vi "EFDUV Example Read Ultimus V Dispense Parameters.vi"(0 "VISA resource name":refnum<visa-resource-name>="COM1", 5 "Serial Configuration":T1={"Baud Rate "=115200, "Parity "=0, "Data Bits "=8, "Stop Bits"=10} {"Stop Bits" items=["1.0"=10, "1.5"=15, "2.0"=20]; "Data Bits" items=["7"=7, "8"=8]; "Parity" items=["None", "Odd", "Even"]; "Baud Rate" items=["9600"=9600, "19200"=19200, "38400"=38400, "115200"=115200]}) -> (1 "CLOCK":string caption="Start", 2 "SHOT":i32 caption="Start" format="%07.0f", 3 "TRIGGER":dbl caption="Start", 4 "START":i32 caption="Start", 6 "END":i32 caption="Start", 8 "STEADY LABEL":string caption="Start", 10 "PRES":dbl caption="Start", 12 "MEM":i32 caption="Start", 13 "AI":string caption="Start", 15 "VAC":dbl caption="Start")   [LabVIEW 2016]
doc: "Reads the dispense parameters that the Ultimus V dispenser is currently set to. This vi reads, the set parameters that are currently on the Ultimus V home screen."
uses:
  EFD Ultimus V.lvlib
panel:
  out "TIME":dbl caption="Start"
  out "Pressure_Units":string="psi" caption="Start"
  out "Vacuum Units":string="\"H20" caption="Start"
  in  "Tab Control 2":enum32{"Read Ultimus V Unit"}(tab)
  # "1.Select the Serial Comm \nPort Associated with the \nUltimus V unit"
  # "2.Select the Configuration Settings.\nThe default settings are 115200,None,8,1"
  # "3.Click the Run Button to Update the Screen."
  # "STRT :"
  # "END   :"
  # "SHOT :"
  # "AI     :"
  # "TRIG :"
  # "MEM  :"
  # "TIME :"
  # "PRES :"
  # "VAC  :"
  # "www.efd-inc.com"
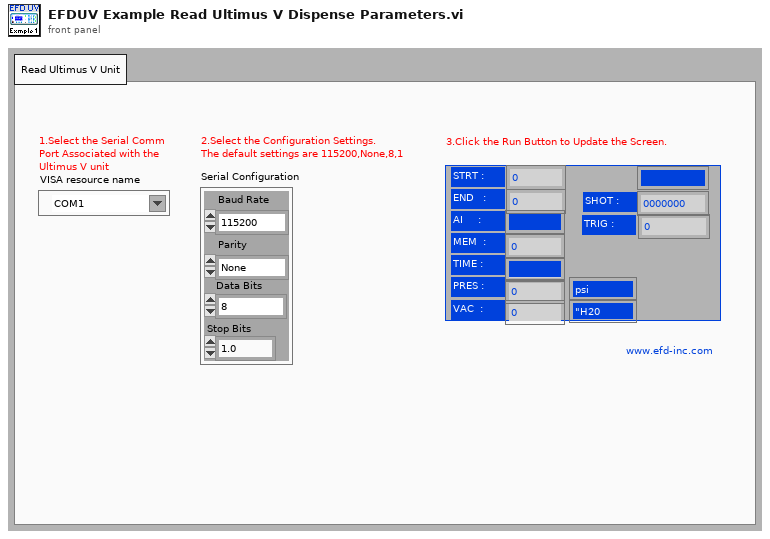
[diagram p1: front panel]
types:
  T1 = cluster{"Baud Rate ":u32, "Parity ":u16, "Data Bits ":u16, "Stop Bits":u16}
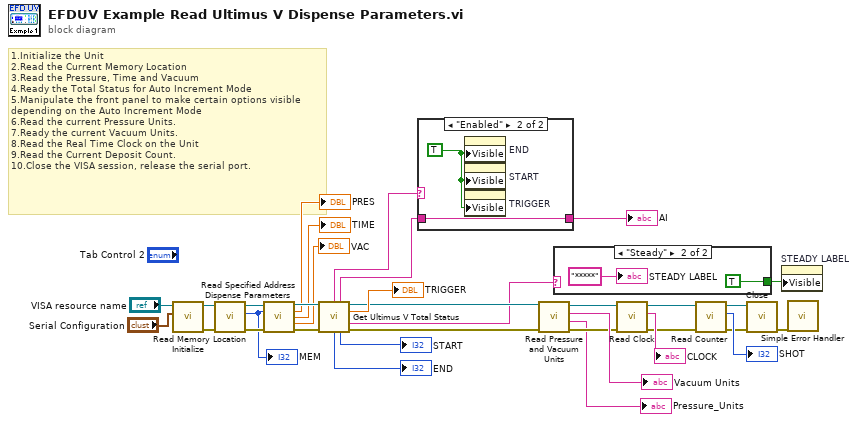
[diagram p0: block diagram]
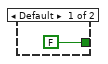
[diagram p2: hidden frame]
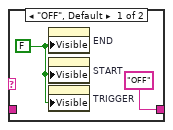
[diagram p3: hidden frame]
diagram:
  # "1.Initialize the Unit\n2.Read the Current Memory Location\n3.Read the Pressure, Time and Vacuum\n4.Ready the Total Status for Auto Increment Mode\n5.Manipulate the front panel to make certain options visible\ndepending on the Auto Increment Mode\n6.Read the current Pressure Units.\n7.Ready the current Vacuum Units.\n8.Read the Real Time Clock on the Unit\n9.Read the Current Deposit Count.\n10.Close the VISA session, release the serial port."
  n1 = call "Initialize.vi"("Serial Configuration"="Serial Configuration", "VISA resource name"="VISA resource name") -> ("error out"=w31:errorcluster, "VISA resource name out"=w29:refnum<visa-resource-name>)  [unwired: 8 in]
  n2 = call "Read Memory Location.vi"("error in (no error)"=w31, "VISA resource name"=w29) -> ("error out"=w30:errorcluster, "Memory Location"=w25:i32, "VISA resource name out"=w28:refnum<visa-resource-name>)  [unwired: 7 in]
  "MEM" <- w25
  n3 = call "Read Specified Address Dispense Parameters.vi"("VISA resource name"=w28, "Memory Location (ccc)"=w25, "error in (no error)"=w30) -> ("VISA resource name out"=w26:refnum<visa-resource-name>, "Pressure"=→"PRES":dbl, "Dispense Time"=→"TIME":dbl, "Vacuum"=→"VAC":dbl, "error out"=w27:errorcluster)  [unwired: 8 in]
  n4 = call "Get Ultimus V Total Status.vi"("VISA resource name"=w26, "error in (no error)"=w27) -> ("AI Mode Status"=w6:string, "AI Mode Function"=w5:string, "VISA resource name out"=w21:refnum<visa-resource-name>, "Trigger Value"=→"TRIGGER":dbl, "Dispense Mode"=w10:string, "AI End Address"=→"END":i32, "AI Start Address"=→"START":i32, "error out"=w22:errorcluster)  [unwired: 5 in, 1 out]
  n5 = case shown="\"Enabled\"" w6 {
    tunnel: ["OFF" ("AI") w37] -> w15
    tunnel: w5 -> [_ w37]
    frame "OFF", Default {
      w34 = FALSE ("Visible")
      n6 = property on="END" class="DigNum (strict)"("Visible"=w34) -> ()  [unwired: 2 in, 2 out]
      n7 = property on="START" class="DigNum (strict)"("Visible"=w34) -> ()  [unwired: 2 in, 2 out]
      n8 = property on="TRIGGER" class="DigNum (strict)"("Visible"=w34) -> ()  [unwired: 2 in, 2 out]
    }
    frame "Enabled" {
      w36 = TRUE ("Visible")
      n9 = property on="END" class="DigNum (strict)"("Visible"=w36) -> ()  [unwired: 2 in, 2 out]
      n10 = property on="START" class="DigNum (strict)"("Visible"=w36) -> ()  [unwired: 2 in, 2 out]
      n11 = property on="TRIGGER" class="DigNum (strict)"("Visible"=w36) -> ()  [unwired: 2 in, 2 out]
    }
  }
  "AI" <- w15
  n12 = call "Read Pressure and Vacuum Units.vi"("error in (no error)"=w22, "VISA resource name"=w21) -> ("error out"=w4:errorcluster, "Pressure Units"=→"Pressure_Units":string, "Vacuum Units"=→"Vacuum Units":string, "VISA resource name out"=w3:refnum<visa-resource-name>)  [unwired: 6 in]
  n13 = case shown="\"Steady\"" w10 {
    tunnel: [FALSE ("Visible") TRUE ("Visible")] -> w9
    frame Default {
    }
    frame "Steady" {
      "STEADY LABEL" <- "*****" ("STEADY LAEL")
    }
  }
  n14 = call "Read Clock.vi"("error in (no error)"=w4, "VISA resource name"=w3) -> ("error out"=w18:errorcluster, "Clock Reading"=→"CLOCK":string, "VISA resource name out"=w17:refnum<visa-resource-name>)  [unwired: 7 in]
  n15 = call "Read Counter.vi"("error in (no error)"=w18, "VISA resource name"=w17) -> ("error out"=w12:errorcluster, "Deposit Counter"=→"SHOT":i32, "VISA resource name out"=w11:refnum<visa-resource-name>)  [unwired: 7 in]
  n16 = call "Close.vi"("error in (no error)"=w12, "VISA resource name"=w11) -> ("error out"=w1:errorcluster)  [unwired: 9 in]
  n17 = property on="STEADY LABEL" class="Str"("Visible"=w9) -> ()  [unwired: 2 in, 2 out]
  n18 = call <vilib>:"Simple Error Handler.vi"("error in (no error)"=w1) -> ()  [unwired: 4 in, 5 out]
